vi "Display.vi"(8 "error in":errorcluster, 11 "Popup in":refnum<class "Popup.lvclass">) -> (0 "error out":errorcluster, 3 "Popup out":refnum<class "Popup.lvclass">)   [LabVIEW 2021, in "Pop-Up.lvlib" / "Popup.lvclass"]
doc: "This is the override method required for each child of the pop up class. It is the pop up that will display to the user.\n\nTo extend this function, create a child class of the pop up class. Then create an override method for this VI. <b>Display.vi</b> is a protected function, therefore it cannot be called in a main application. This VI must be called by a caller function. See one of the standard pop-ups for a setup example.\n\n<b>Code Developed By:</b> +\nDaniel Coons +\nhttps://github.com/danielcoons/tsc-pop-up"
uses:
  Popup.lvclass
  Popup.lvclass/Popup.ctl
  Data Member Access/Read Theme.vi
  Theme/Theme.lvclass
  user32.dll
panel:
  out "message":string
  out "header":bool
  out "2D Picture":picture
  # "This VI displays the popup"
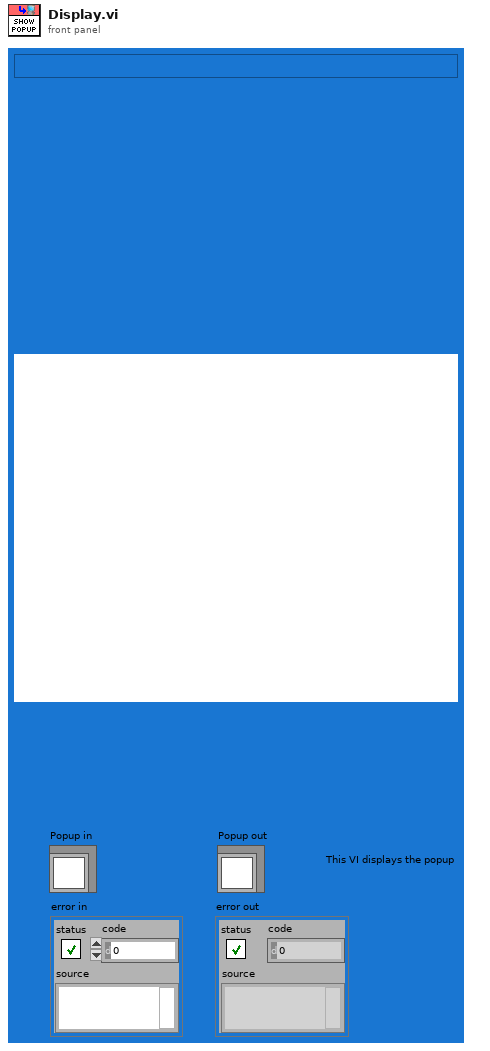
[diagram p1: front panel]
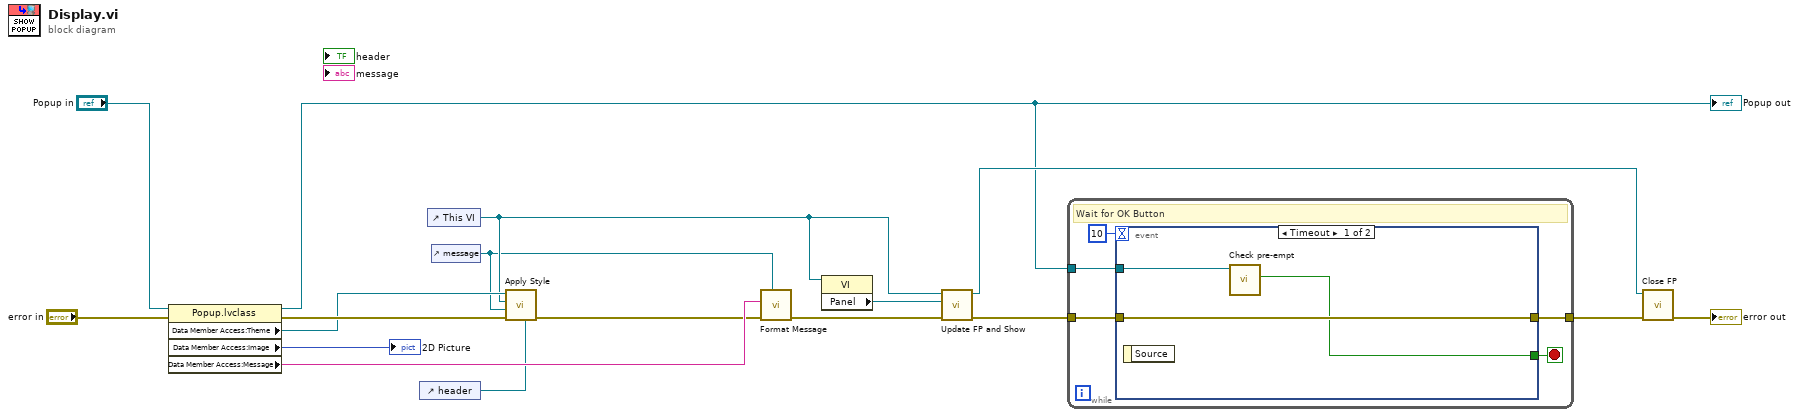
[diagram p0: block diagram]
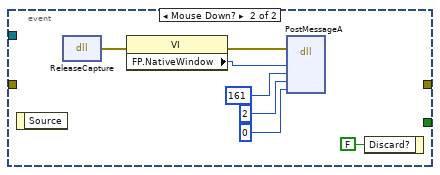
[diagram p2: hidden frame]
diagram:
  n1 = property class="Popup.lvclass"(reference="Popup in", error in="error in") -> (reference out=w2:refnum<class "Popup.lvclass">, error out=w17:errorcluster, "Data Member Access:Theme"=w9:refnum<class "Theme.lvclass">, "Data Member Access:Image"=→"2D Picture":picture, "Data Member Access:Message"=w12:string)
  "Popup out" <- w2
  n2 = control-ref of="header"() -> (w6:refnum<vi>)
  n3 = control-ref of="This VI"() -> (w8:refnum<vi>)
  n4 = control-ref of="message"() -> (w7:refnum<vi>)
  n5 = call "Apply Style.vi"("header ref"=w6, "error in"=w17, "message ref"=w7, "pop up ref"=w8, "Theme in"=w9) -> ("error out"=w10:errorcluster)  [unwired: 5 in, 1 out]
  n6 = call "Format Message.vi"("formatted string"=w7, "error in"=w10, "String Input"=w12) -> ("error out"=w11:errorcluster)  [unwired: 7 in, 1 out]
  n7 = property class="VI"(reference=w8) -> ("Panel"=w15:refnum<vi>)  [unwired: 1 in, 2 out]
  n8 = call "Update FP and Show.vi"("error in (no error)"=w11, "Panel Ref"=w15, "VI in"=w8) -> ("error out"=w14:errorcluster, "VI out"=w13:refnum<vi>)  [unwired: 7 in]
  n9 = while {
    tunnel: [w20] -> w16
    tunnel: w14 -> [w21]
    tunnel: w2 -> [w18]
    stop <- w22 stop-if-true
    # "Wait for OK Button"
    n10 = event shown="[0] Timeout" {
      selector: _ -> [_ _]
      dyn-events: _ -> [_ _]
      timeout: 10 -> [_ _]
      tunnel: [w23 _] -> w22
      tunnel: w21 -> [w25 _]
      tunnel: [w25 _] -> w20
      tunnel: w18 -> [w24 _]
      event Timeout {
        n11 = event-data() -> ()  [unwired: 1 in, 1 out]
        n12 = call "Check pre-empt.vi"("_Popup in"=w24) -> ("Pre-empted?"=w23:bool)  [unwired: 8 in, 2 out]
      }
      event Mouse Down? {
        n13 = event-data() -> ()  [unwired: 1 in, 1 out]
        n14 = dll-call lib="user32.dll" fn="ReleaseCapture"() -> (error out=w30:errorcluster)  [unwired: 4 in, 1 out]
        n15 = property class="VI"(error in=w30) -> (error out=w31:errorcluster, "FP.NativeWindow"=w32:u64)  [unwired: 1 in, 1 out]
        n16 = dll-call lib="user32.dll" fn="PostMessageA"(error in=w31, "hWnd"=w32, "Msg"=161, "wParam"=2, "lParam"=0) -> ()  [unwired: 7 in, 2 out]
        n17 = event-data("Discard?"=FALSE) -> ()  [unwired: 1 in, 1 out]
      }
    }
  }
  n18 = call "Close FP.vi"("error in (no error)"=w16, "VI in"=w13) -> ("error out"=→"error out":errorcluster)  [unwired: 9 in]
